vi "Read.vi"(8 "error in (no error)":errorcluster, 11 "Queue in":refnum<class "Queue.lvclass">) -> (0 "error out":errorcluster, 2 "DATA":T1, 3 "Queue out":refnum<class "Queue.lvclass">)   [LabVIEW 2020, in "Queue.lvclass"]
uses:
  Queue.lvclass
  Queue.lvclass/Queue.ctl
  Accessors/Read/Read DATA.vi
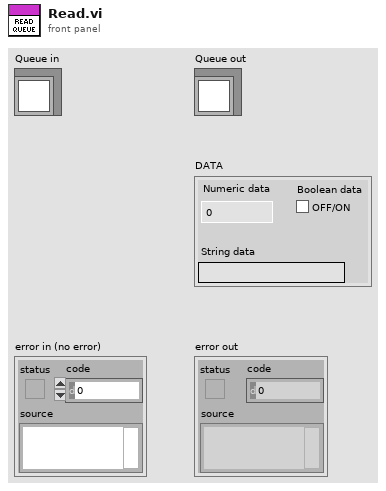
[diagram p1: front panel]
types:
  T1 = cluster{"Numeric data":dbl, "String data":string, "Boolean data":bool}
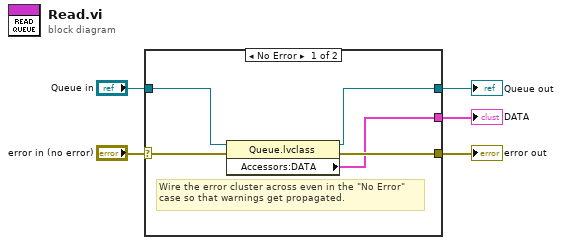
[diagram p0: block diagram]
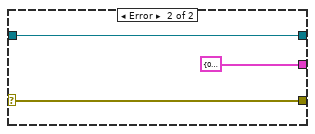
[diagram p2: hidden frame]
diagram:
  n1 = case shown="No Error" "error in (no error)" {
    selector: "error in (no error)" -> [w10 w13]
    tunnel: [w7 w13] -> w4
    tunnel: [w8 w12] -> w2
    tunnel: "Queue in" -> [w9 w12]
    tunnel: [w6 T1 {"Numeric data"=0.0, "String data"="", "Boolean data"=FALSE} ("Accessors:DATA")] -> w1
    frame No Error {
      # "Wire the error cluster across even in the \"No Error\"\ncase so that warnings get propagated."
      n2 = property class="Queue.lvclass"(reference=w9, error in=w10) -> (reference out=w8:refnum<class "Queue.lvclass">, error out=w7:errorcluster, "Accessors:DATA"=w6:T1)
    }
    frame Error {
    }
  }
  "error out" <- w4
  "Queue out" <- w2
  "DATA" <- w1
